vi "RDS Child Receive Message.vi"(8 "error in (no error)":errorcluster, 10 "RDS Message":refnum<class "RDS Message.lvclass">, 11 "RDS Local Remote Actor in":refnum<class "RDS Local Remote Actor.lvclass">) -> (0 "error out":errorcluster, 3 "RDS Local Remote Actor out":refnum<class "RDS Local Remote Actor.lvclass">)   [LabVIEW 2015, in "RDS Local Remote Actor.lvlib" / "RDS Local Remote Actor.lvclass"]
uses:
  RDS Local Remote Actor.lvclass
  Libraries/RDS Framework/RDS Message Class/RDS Message.lvclass
  Libraries/RDS Framework/RDS Message Class/RDS Message.lvclass/RDS Message.ctl
  Libraries/RDS Child Messages/Controller Message/Controller Message.lvclass
  Libraries/RDS Child Messages/Controller Message/Controller Message.lvclass/Controller Message.ctl
  RDS Local Remote Actor.lvclass/RDS Local Remote Actor.ctl
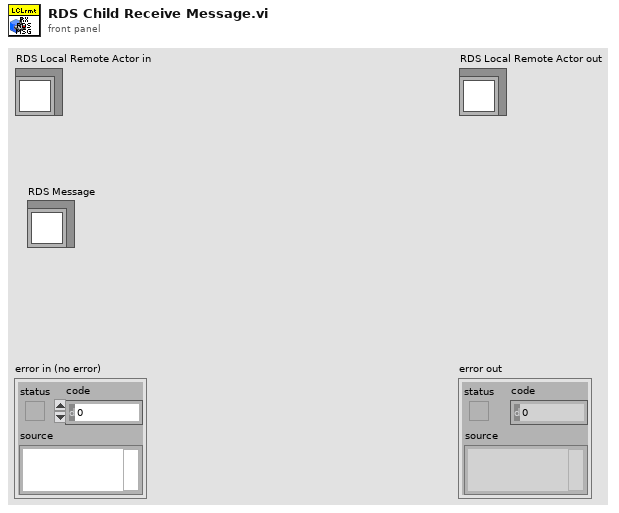
[diagram p1: front panel]
types:
  T1 = typedef "RDS Child Messages.lvlib/RDS Message ID.ctl" = enum16{"RDS Hello World", "String Message", "AIP_Status", "AIP_Command", "GPS_Data", "MCB_Command", "MCB_Status", "Compass_Data", "Depth_Data", "Battery_Data", "Contoller_State", "Set_Mag_Dev", "BTB_Shutdown", "State_Sample_Request", "State_Sample", "PID_Gains_Set", "Helm_Limiter_Set", "Helm_Heading_Command", "Helm_Steering_Command", "Helm_Status", "Controller_Message", "AIP_Set_Min_Depth", "Mission_Controller_State", "Mission_Upload", "Mission_Set_Op_and_Run", "Mission_Settings_Set"}
  T2 = typedef "RDS Controller Actor.lvlib/Controller.ctl" = enum16{"Idle", "Local Remote Control", "Shore Remote Control", "Mission Control"}
  T3 = typedef "RDS Child Messages.lvlib/Controller Message.lvclass/Controller Message Type.ctl" = enum16{"Control Relinquish Request", "Control Relinquish Command", "Control Request", "Control Granted"}
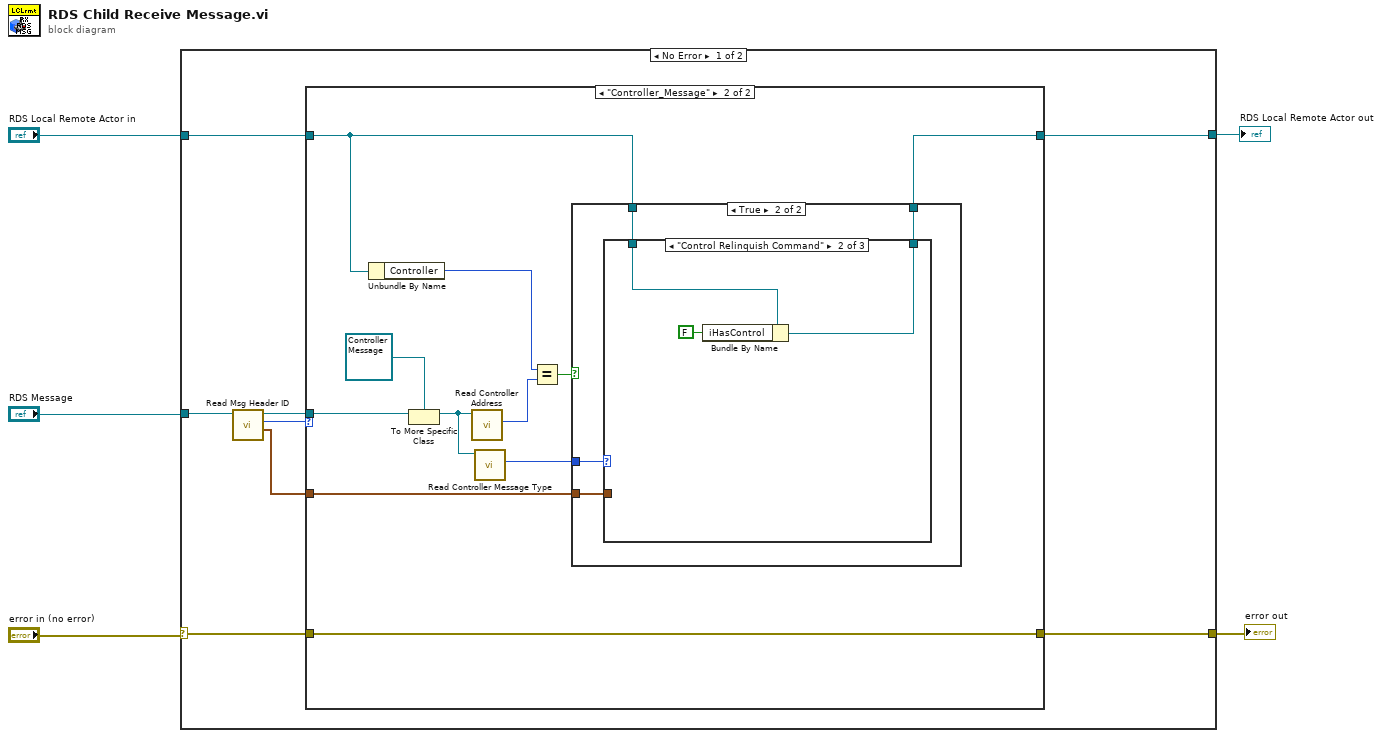
[diagram p0: block diagram]
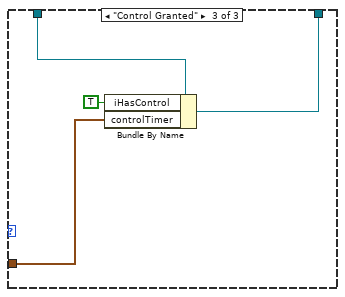
[diagram p5: hidden frame]
diagram:
  n1 = case shown="No Error" "error in (no error)" {
    selector: "error in (no error)" -> [w9 w40]
    tunnel: "RDS Message" -> [w13 _]
    tunnel: "RDS Local Remote Actor in" -> [w7 w41]
    tunnel: [w8 w41] -> w1
    tunnel: [w10 w40] -> w5
    frame No Error {
      n2 = call "Read Msg Header ID.vi"("RDS Message in"=w13) -> ("Time Stamp"=w6:timestamp, "Msg ID"=w12:T1, "RDS Message out"=w11:refnum<class "RDS Message.lvclass">)  [unwired: 6 in, 2 out]
      n3 = case shown="\"Controller_Message\"" w12 {
        tunnel: w11 -> [_ w26]
        tunnel: [w15 w25] -> w10
        tunnel: w9 -> [w15 w25]
        tunnel: w7 -> [w14 w19]
        tunnel: [w14 w21] -> w8
        tunnel: w6 -> [_ w20]
        frame "RDS Hello World", Default {
        }
        frame "Controller_Message" {
          n4 = Unbundle By Name(w19) -> ("Controller"=w17:T2)
          n5 = To More Specific Class(target class=refnum<class "Controller Message.lvclass"> refnum ("RDS Child Messages.lvlib:Controller Message.lvclass"), reference=w26) -> (specific class reference=w23:refnum<class "Controller Message.lvclass">)  [unwired: 1 in, 1 out]
          n6 = call "Read Controller Address.vi"("Controller Message in"=w23) -> ("Controller"=w18:T2)  [unwired: 8 in, 2 out]
          n7 = call "Read Controller Message Type.vi"("Controller Message in"=w23) -> ("Controller Message Type"=w22:T3)  [unwired: 8 in, 2 out]
          n8 = Equal?(x=w17, y=w18) -> (x = y?=w16:bool)
          n9 = case shown="True" w16 {
            tunnel: w22 -> [_ w31]
            tunnel: w19 -> [w27 w30]
            tunnel: [w27 w29] -> w21
            tunnel: w20 -> [_ w28]
            frame False {
            }
            frame True {
              n10 = case shown="\"Control Relinquish Command\"" w31 {
                tunnel: w30 -> [w32 w35 w39]
                tunnel: [w32 w33 w37] -> w29
                tunnel: w28 -> [_ _ w36]
                frame "Control Relinquish Request", Default {
                  # "not for us"
                }
                frame "Control Relinquish Command" {
                  n11 = Bundle By Name(cluster=w35, "iHasControl"=FALSE) -> (w33:refnum<class "RDS Local Remote Actor.lvclass">)
                }
                frame "Control Granted" {
                  n12 = Bundle By Name(cluster=w39, "iHasControl"=TRUE, "controlTimer"=w36) -> (w37:refnum<class "RDS Local Remote Actor.lvclass">)
                }
              }
            }
          }
        }
      }
    }
    frame Error {
    }
  }
  "error out" <- w5
  "RDS Local Remote Actor out" <- w1
